vi "Boolean to Listbox Symbol.vi"(7 "Boolean":bool) -> (8 "Symbol":i32)   [LabVIEW 2020]
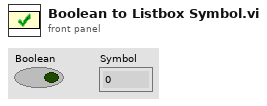
[diagram p1: front panel]
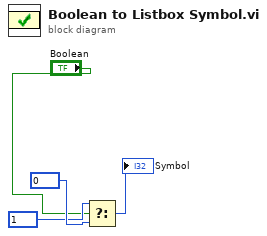
[diagram p0: block diagram]
diagram:
  n1 = Select(t=1, s="Boolean", f=0) -> (s? t:f=→"Symbol":i32)
